vi "combine_dataset.vi"(6 "Class Name":u16(ring) items=["bump", "hair", "cut"], 8 "Bounding Boxes In":T1(array[cluster]), 9 "Data In":string[][](array[string]), 11 "Image Directory":path) -> (1 "Data Out":string[][](array[string]))   [LabVIEW 2019]
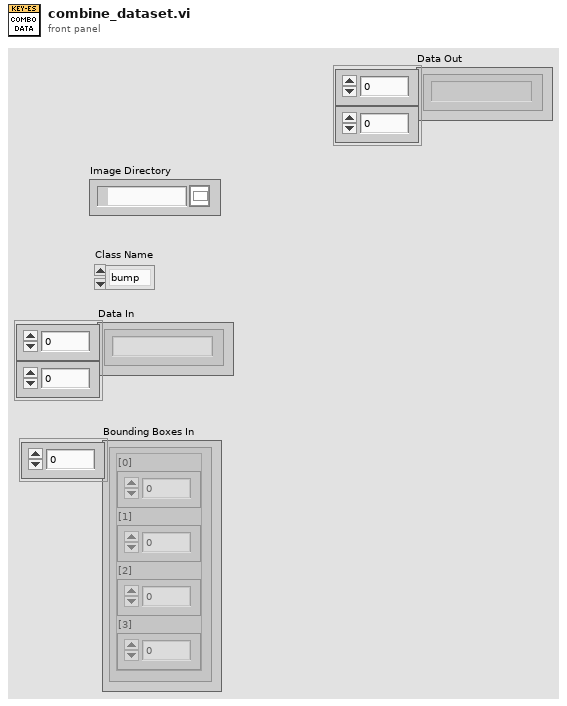
[diagram p1: front panel]
types:
  T1 = cluster{"[0]":i32, "[1]":i32, "[2]":i32, "[3]":i32}[]
  T2 = cluster{"[0]":i32, "[1]":i32, "[2]":i32, "[3]":i32}
  T3 = cluster{string, string, string, string, string, string}
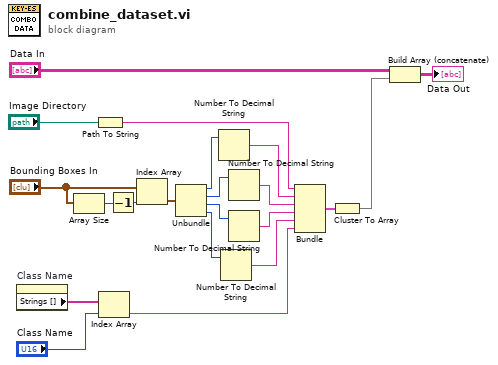
[diagram p0: block diagram]
diagram:
  n1 = property on="Class Name" class="Ring (strict)"() -> ("Strings []"=w5:string[])  [unwired: 2 in, 2 out]
  n2 = Array Size(array="Bounding Boxes In") -> (size(s)=w11:i32)
  n3 = Path To String(path="Image Directory") -> (string=w21:string)
  n4 = Index Array(array=w5, index="Class Name") -> (element=w4:string)
  n5 = Decrement(x=w11) -> (x-1=w10:i32)
  n6 = Index Array(array="Bounding Boxes In", index=w10) -> (element=w8:T2)
  n7 = Unbundle(w8) -> ("[0]"=w12:i32, "[1]"=w14:i32, "[2]"=w16:i32, "[3]"=w18:i32)
  n8 = Number To Decimal String(number=w12) -> (decimal integer string=w13:string)  [unwired: 1 in]
  n9 = Number To Decimal String(number=w18) -> (decimal integer string=w19:string)  [unwired: 1 in]
  n10 = Number To Decimal String(number=w14) -> (decimal integer string=w15:string)  [unwired: 1 in]
  n11 = Number To Decimal String(number=w16) -> (decimal integer string=w17:string)  [unwired: 1 in]
  n12 = Bundle(w21, w13, w15, w17, w19, w4) -> (w20:T3)  [unwired: 1 in]
  n13 = Cluster To Array(cluster=w20) -> (array=w2:string[])
  n14 = Build Array (concatenate)("Data In", w2) -> (→"Data Out":string[][])
